vi "Simple image acquisition mono - events.vi"() -> ()   [LabVIEW 2015]
uses:
  C:/code/Host/Installer/Scientific Camera Interfaces/LabVIEW/32_bit/Library_X86/Thorlabs.TSI.TLCameraInterfaces.dll
  32_bit/Library_X86/Thorlabs.TSI.TLCameraInterfaces.dll
  SubVIs/Parameters Get & Set/Set Parameters/Set ExposureTime_us.vi
  SubVIs/Parameters Get & Set/Set Parameters/Set OperationMode.vi
  SubVIs/Parameters Get & Set/Set Parameters/Set FramesPerTrigger_zeroForUnlimited.vi
panel:
  in  "Exposure (ms)":u32=100
  out "Camera Diagnostics Message":string
  in  "stop":bool
  out "FrameNumber":i32
  out "Intensity Graph Mono or Blue":u16[][](graph)
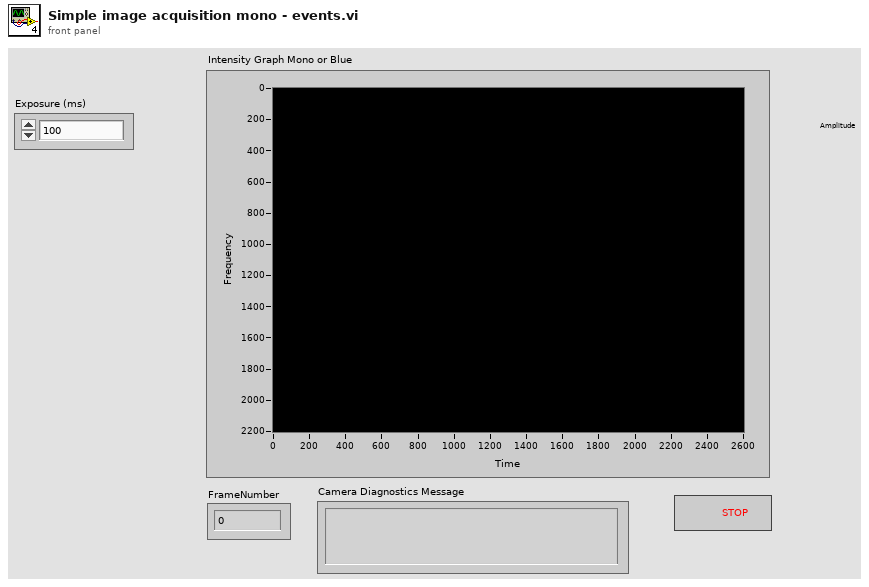
[diagram p1: front panel]
types:
  T1 = cluster{"Thorlabs.TSI.TLCameraInterfaces.ITLCamera":refnum<k24>, "FrameNumber":refnum<vi>, "Intensity Graph":refnum<vi>}
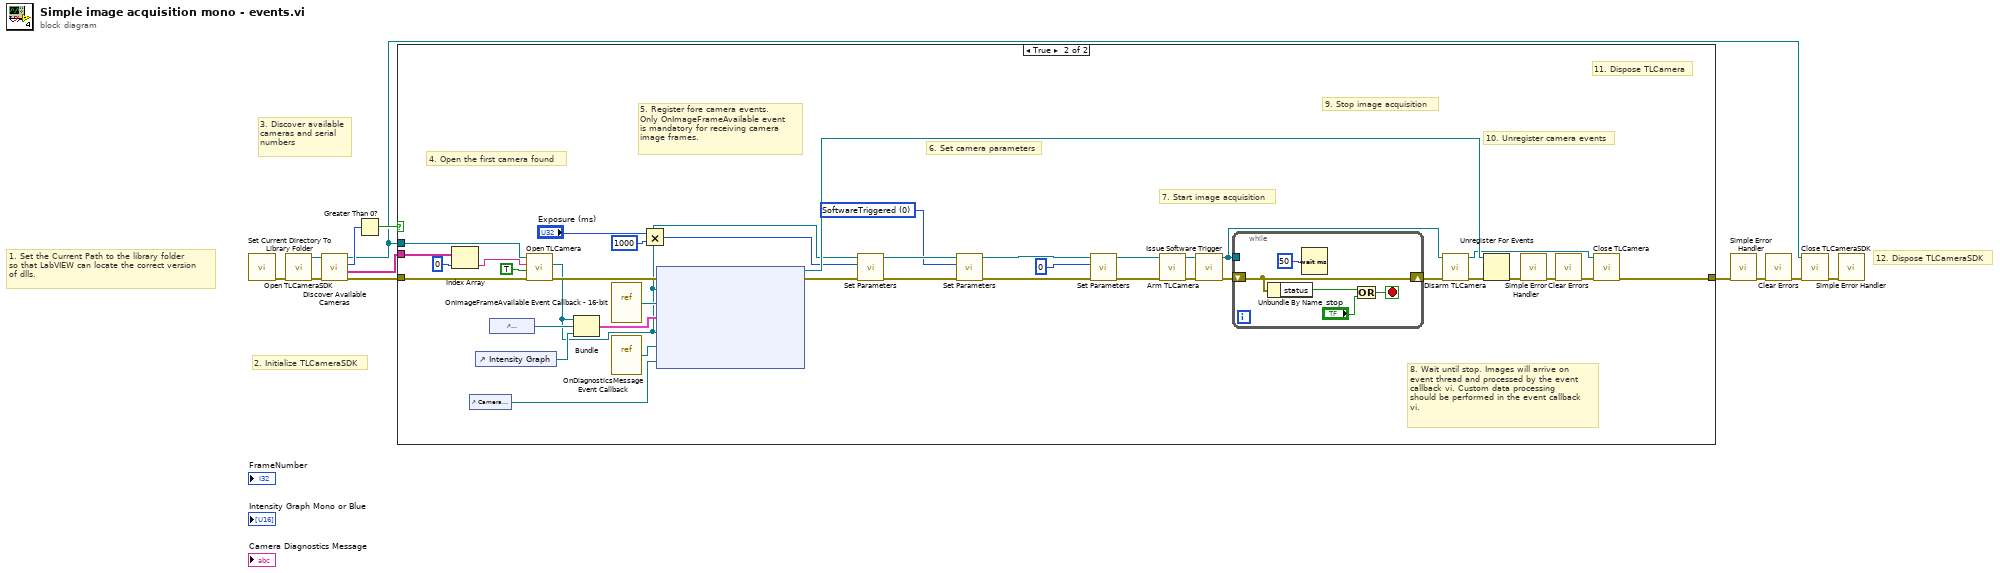
[diagram p0: block diagram]
diagram:
  # "1. Set the Current Path to the library folder\nso that LabVIEW can locate the correct version\nof dlls."
  # "12. Dispose TLCameraSDK"
  # "3. Discover available\ncameras and serial \nnumbers"
  # "2. Initialize TLCameraSDK"
  n1 = call "Set Current Directory To Library Folder.vi"() -> ("error out"=w6:errorcluster)  [unwired: 11 in]
  n2 = call "Open TLCameraSDK.vi"("error in (no error)"=w6) -> ("error out"=w5:errorcluster, "Thorlabs.TSI.TLCameraInterfaces.ITLCameraSDK"=w4:refnum<k24>)  [unwired: 9 in]
  n3 = call "Discover Available Cameras.vi"("error in (no error)"=w5, "Thorlabs.TSI.TLCameraInterfaces.ITLCameraSDK"=w4) -> ("error out"=w10:errorcluster, "Serial Numbers"=w9:string[], "Number of Cameras"=w12:i32, "Thorlabs.TSI.TLCameraInterfaces.ITLCameraSDK"=w8:refnum<k24>)  [unwired: 6 in]
  n4 = Greater Than 0?(x=w12) -> (x > 0?=w11:bool)
  n5 = case shown="True" w11 {
    tunnel: w10 -> [w13 w37]
    tunnel: w9 -> [_ w51]
    tunnel: w8 -> [_ w40]
    tunnel: [w13 w28] -> w3
    frame False {
    }
    frame True {
      w19 = 0 items=["SoftwareTriggered", "HardwareTriggered", "Bulb", "Reserved1", "Reserved2"] ("OperationMode")
      # "11. Dispose TLCamera"
      # "10. Unregister camera events"
      # "9. Stop image acquisition"
      # "8. Wait until stop. Images will arrive on \nevent thread and processed by the event \ncallback vi. Custom data processing \nshould be performed in the event callback\nvi."
      # "7. Start image acquisition"
      # "6. Set camera parameters"
      # "5. Register fore camera events.\nOnly OnImageFrameAvailable event\nis mandatory for receiving camera\nimage frames."
      # "4. Open the first camera found"
      n6 = Index Array(array=w51, index=0) -> (element=w38:string)
      n7 = control-ref of="Camera Diagnostics Message"() -> (w44:refnum<vi>)
      n8 = control-ref of="Intensity Graph"() -> (w48:refnum<vi>)
      n9 = control-ref of="FrameNumber"() -> (w49:refnum<vi>)
      n10 = call "Open TLCamera.vi"("error in (no error)"=w37, "isDiagnosticsMessagesEnabled"=TRUE, "Camera serial number"=w38, "Thorlabs.TSI.TLCameraInterfaces.ITLCameraSDK"=w40) -> ("error out"=w36:errorcluster, "Thorlabs.TSI.TLCameraInterfaces.ITLCamera"=w14:refnum<k24>)  [unwired: 5 in, 1 out]
      n11 = Bundle("Thorlabs.TSI.TLCameraInterfaces.ITLCamera"=w14, "FrameNumber"=w49, "Intensity Graph"=w48) -> (w47:T1)  [unwired: 1 in]
      n12 = vi-ref "OnImageFrameAvailable Event Callback - 16-bit.vi"() -> ("vi reference"=w46:refnum<vi>)
      n13 = vi-ref "OnDiagnosticsMessage Event Callback.vi"() -> ("vi reference"=w43:refnum<vi>)
      n14 = Multiply(x="Exposure (ms)", y=u32 1000) -> (x*y=w27:u32)
      n15 = node(w36, w14, w46, w47, w14, w43, w44) -> (w45:refnum<k27>, w15:errorcluster)  [unwired: 1 in]
      n16 = call-poly "Set Parameters.vi"("error in (no error)"=w15, "ExposureTime_us"=w27, "Thorlabs.TSI.TLCameraInterfaces.ITLCamera"=w14) -> ("error out"=w25:errorcluster, "Thorlabs.TSI.TLCameraInterfaces.ITLCamera"=w26:refnum<k24>)  [unwired: 7 in]
      n17 = call-poly "Set Parameters.vi"("error in (no error)"=w25, "OperationMode"=w19, "Thorlabs.TSI.TLCameraInterfaces.ITLCamera"=w26) -> ("error out"=w20:errorcluster, "Thorlabs.TSI.TLCameraInterfaces.ITLCamera"=w24:refnum<k24>)  [unwired: 7 in]
      n18 = call-poly "Set Parameters.vi"("error in (no error)"=w20, "FramesPerTrigger_zeroForUnlimited"=u32 0 ("FramesPerTriggerOrZeroForUnlimited"), "Thorlabs.TSI.TLCameraInterfaces.ITLCamera"=w24) -> ("error out"=w22:errorcluster, "Thorlabs.TSI.TLCameraInterfaces.ITLCamera"=w23:refnum<k24>)  [unwired: 7 in]
      n19 = call "Arm TLCamera.vi"("error in (no error)"=w22, "Thorlabs.TSI.TLCameraInterfaces.ITLCamera"=w23) -> ("error out"=w34:errorcluster, "Thorlabs.TSI.TLCameraInterfaces.ITLCamera"=w35:refnum<k24>)  [unwired: 8 in]
      n20 = call "Issue Software Trigger.vi"("error in (no error)"=w34, "Thorlabs.TSI.TLCameraInterfaces.ITLCamera"=w35) -> ("error out"=w33:errorcluster, "Thorlabs.TSI.TLCameraInterfaces.ITLCamera"=w32:refnum<k24>)  [unwired: 8 in]
      n21 = while {
        tunnel: w32 -> [_]
        shift-right: [w52] -> w31
        shift-left: w33 -> [w52]
        stop <- w55 stop-if-true
        n22 = Unbundle By Name(w52) -> ("status"=w54:bool)
        n23 = Wait (ms)(milliseconds to wait=u32 50) -> ()  [unwired: 1 out]
        n24 = Or(x=w54, y="stop") -> (x .or. y?=w55:bool)
      }
      n25 = call "Disarm TLCamera.vi"("error in (no error)"=w31, "Thorlabs.TSI.TLCameraInterfaces.ITLCamera"=w32) -> ("error out"=w30:errorcluster, "Thorlabs.TSI.TLCameraInterfaces.ITLCamera"=w29:refnum<k24>)  [unwired: 8 in]
      n26 = Unregister For Events(event registration refnum=w45, error in=w30) -> (error out=w18:errorcluster)
      n27 = call <vilib>:"Simple Error Handler.vi"("error in (no error)"=w18) -> ("error out"=w16:errorcluster)  [unwired: 4 in, 4 out]
      n28 = call <vilib>:"Clear Errors.vi"("error in (no error)"=w16) -> ("error out"=w17:errorcluster)  [unwired: 5 in, 1 out]
      n29 = call "Close TLCamera.vi"("error in (no error)"=w17, "Thorlabs.TSI.TLCameraInterfaces.ITLCamera"=w29) -> ("error out"=w28:errorcluster)  [unwired: 9 in]
    }
  }
  n30 = call <vilib>:"Simple Error Handler.vi"("error in (no error)"=w3) -> ("error out"=w1:errorcluster)  [unwired: 4 in, 4 out]
  n31 = call <vilib>:"Clear Errors.vi"("error in (no error)"=w1) -> ("error out"=w2:errorcluster)  [unwired: 5 in, 1 out]
  n32 = call "Close TLCameraSDK.vi"("error in (no error)"=w2, "Thorlabs.TSI.TLCameraInterfaces.ITLCameraSDK"=w8) -> ("error out"=w7:errorcluster)  [unwired: 9 in]
  n33 = call <vilib>:"Simple Error Handler.vi"("error in (no error)"=w7) -> ()  [unwired: 4 in, 5 out]
